vi "Read ALL Auto Drive constants.vi"(8 "error in (no error)":errorcluster) -> (0 "error out":errorcluster, 3 "All Drive Constants":T1)   [LabVIEW 2013]
uses:
  All Auto Drive constants.ctl
  Drive auto constants.ctl
  Drive Code/Auto Transmission Code/All Shifter Constants.ctl
  Drive Code/Auto Transmission Code/Shift Constants.ctl
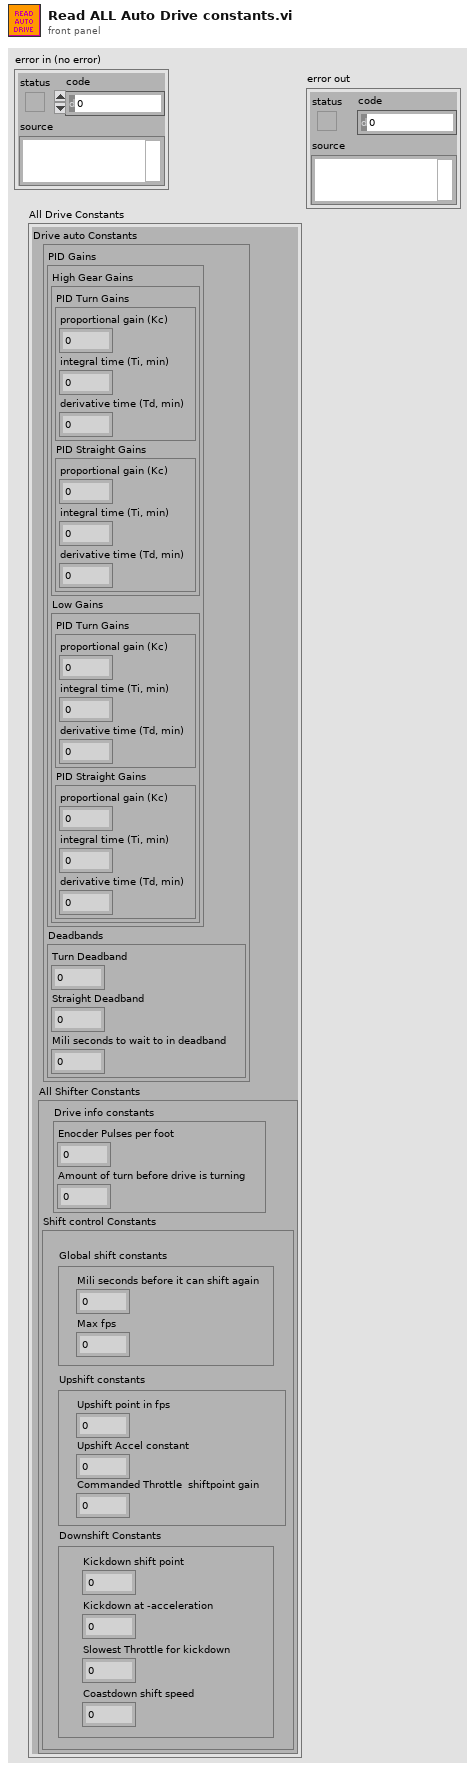
[diagram p1: front panel]
types:
  T1 = typedef "All Auto Drive constants.ctl" = cluster{"Drive auto Constants":T2, "All Shifter Constants":T3}
  T2 = typedef "Drive auto constants.ctl" = cluster{"PID Gains":cluster{"High Gear Gains":cluster{"PID Turn Gains":cluster{"proportional gain (Kc)":dbl, "integral time (Ti, min)":dbl, "derivative time (Td, min)":dbl}, "PID Straight Gains":cluster{"proportional gain (Kc)":dbl, "integral time (Ti, min)":dbl, "derivative time (Td, min)":dbl}}, "Low Gains":cluster{"PID Turn Gains":cluster{"proportional gain (Kc)":dbl, "integral time (Ti, min)":dbl, "derivative time (Td, min)":dbl}, "PID Straight Gains":cluster{"proportional gain (Kc)":dbl, "integral time (Ti, min)":dbl, "derivative time (Td, min)":dbl}}}, "Deadbands":cluster{"Turn Deadband":dbl, "Straight Deadband":dbl, "Mili seconds to wait to in deadband":u32}}
  T3 = typedef "All Shifter Constants.ctl" = cluster{"Drive info constants":cluster{"Enocder Pulses per foot":dbl, "Amount of turn before drive is turning":dbl}, "Shift control Constants":T4}
  T4 = typedef "Shift Constants.ctl" = cluster{"Global shift constants":cluster{"Mili seconds before it can shift again":u32, "Max fps":dbl}, "Upshift constants":cluster{"Upshift point in fps":dbl, "Upshift Accel constant":dbl, "Commanded Throttle  shiftpoint gain":dbl}, "Downshift Constants":cluster{"Kickdown shift point":dbl, "Kickdown at -acceleration":dbl, "Slowest Throttle for kickdown":dbl, "Coastdown shift speed":dbl}}
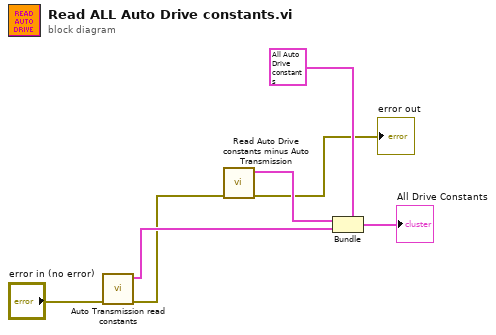
[diagram p0: block diagram]
diagram:
  n1 = call "Auto Transmission read constants.vi"("error in (no error)"="error in (no error)") -> ("error out"=w2:errorcluster, "All Shifter Constants"=w3:T3)  [unwired: 9 in]
  n2 = call "Read Auto Drive constants minus Auto Transmission.vi"("error in (no error)"=w2) -> ("error out"=→"error out":errorcluster, "Auto Drive Constants"=w6:T2)  [unwired: 9 in]
  n3 = Bundle(cluster=T1 {"Drive auto Constants"={"PID Gains"={"High Gear Gains"={"PID Turn Gains"={"proportional gain (Kc)"=0.0, "integral time (Ti, min)"=0.0, "derivative time (Td, min)"=0.0}, "PID Straight Gains"={"proportional gain (Kc)"=0.0, "integral time (Ti, min)"=0.0, "derivative time (Td, min)"=0.0}}, "Low Gains"={"PID Turn Gains"={"proportional gain (Kc)"=0.0, "integral time (Ti, min)"=0.0, "derivative time (Td, min)"=0.0}, "PID Straight Gains"={"proportional gain (Kc)"=0.0, "integral time (Ti, min)"=0.0, "derivative time (Td, min)"=0.0}}}, "Deadbands"={"Turn Deadband"=0.0, "Straight Deadband"=0.0, "Mili seconds to wait to in deadband"=0}}, "All Shifter Constants"={"Drive info constants"={"Enocder Pulses per foot"=0.0, "Amount of turn before drive is turning"=0.0}, "Shift control Constants"={"Global shift constants"={"Mili seconds before it can shift again"=0, "Max fps"=0.0}, "Upshift constants"={"Upshift point in fps"=0.0, "Upshift Accel constant"=0.0, "Commanded Throttle  shiftpoint gain"=0.0}, "Downshift Constants"={"Kickdown shift point"=0.0, "Kickdown at -acceleration"=0.0, "Slowest Throttle for kickdown"=0.0, "Coastdown shift speed"=0.0}}}} ("All Auto Drive constants"), "Drive auto Constants"=w6, "All Shifter Constants"=w3) -> (→"All Drive Constants":T1)
